vi "Settings Dialog.vi"(8 "error in (no error)":errorcluster caption="错误输入（无错误）", 11 "Configuration in":T1={"Hardware Configuration"={"Physical Channel"="", "Maximum Input"=0.0, "Minimum Input"=0.0, "Sample Rate"=0.0, "Number of Samples"=0}, "Analysis Configuration"={"Statistics"=TRUE}, "New Data Behavior"=enum."Replace", "HWInfo"=""} caption="配置输入") -> (0 "error out":errorcluster caption="错误输出", 2 "UI Refresh Needed?":bool caption="需要刷新UI？", 3 "Configuration out":T1={"Hardware Configuration"={"Physical Channel"="", "Maximum Input"=0.0, "Minimum Input"=0.0, "Sample Rate"=0.0, "Number of Samples"=0}, "Analysis Configuration"={"Statistics"=TRUE}, "New Data Behavior"=enum."Replace", "HWInfo"=""} caption="配置输出")   [LabVIEW 2014, in "Acquisitions.lvlib"]
doc: "用于选择用户设置的对话框。"
uses:
  Acquisitions.lvlib
  User Specified Data.ctl
  HW Configuration.ctl
  AcqControls/Analysis Configuration.ctl
  AcqControls/New Data Behavior.ctl
panel:
  in  "采集模块编号":string
  in  "Number of Samples":i32=1000 caption="采样数"
  in  "Sample Rate":dbl=1000.0 caption="采样率"
  in  "Minimum Input":dbl=-10.0 caption="最小输入"
  in  "Maximum Input":dbl=10.0 caption="最大输入"
  in  "Physical Channel":tag="Dev1/ai0:31" caption="物理通道"
  in  "New Data Behavior":u16(ring) caption="新采集到数据时如何操作" items=["替换", "叠加", "添加"]
  in  "Cancel Button":bool caption="取消按钮"
  in  "OK Button":bool caption="确定按钮"
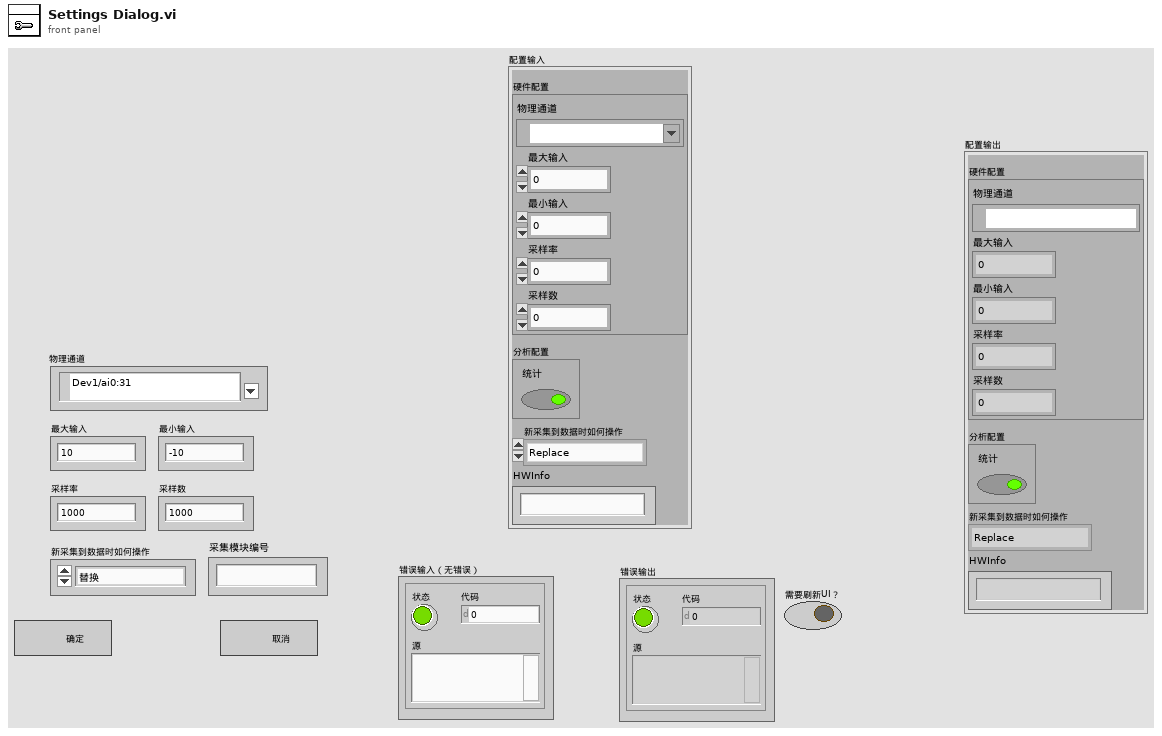
[diagram p1: front panel]
types:
  T1 = typedef "Acquisitions.lvlib/User Specified Data.ctl" = cluster{"Hardware Configuration":T2, "Analysis Configuration":T3, "New Data Behavior":T4, "HWInfo":string}
  T2 = typedef "Acquisitions.lvlib/HW Configuration.ctl" = cluster{"Physical Channel":tag, "Maximum Input":dbl, "Minimum Input":dbl, "Sample Rate":dbl, "Number of Samples":i32}
  T3 = typedef "Acquisitions.lvlib/Analysis Configuration.ctl" = cluster{"Statistics":bool}
  T4 = typedef "Acquisitions.lvlib/New Data Behavior.ctl" = enum16{"Replace", "Overlay", "Append"}
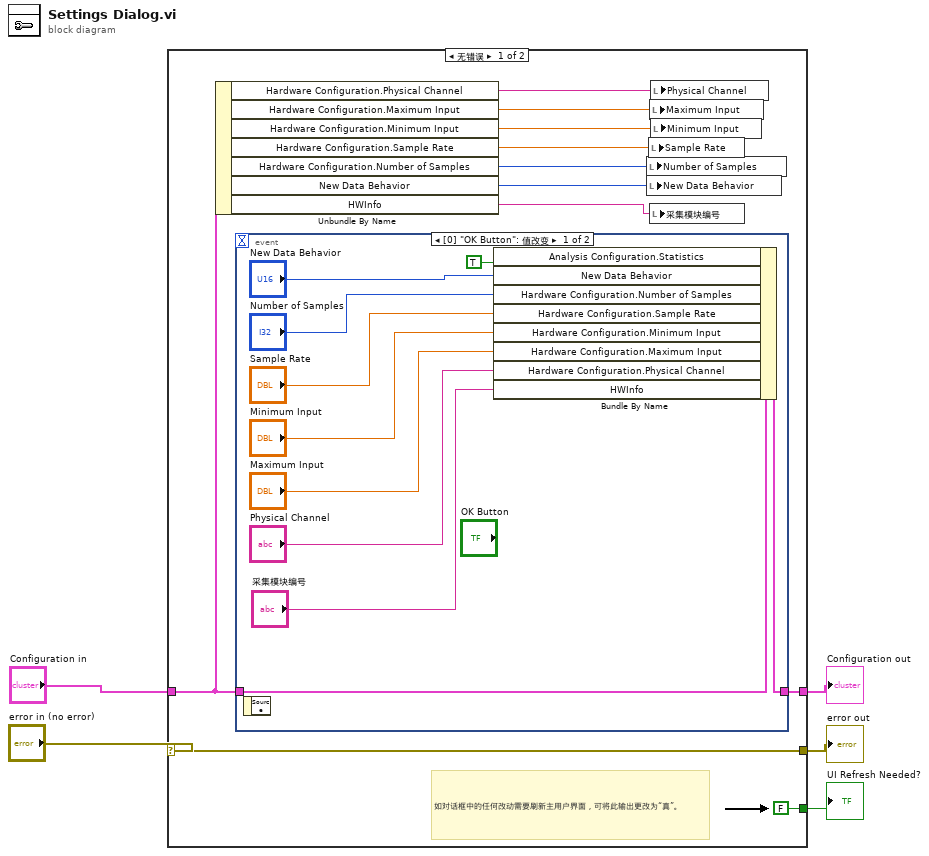
[diagram p0: block diagram]
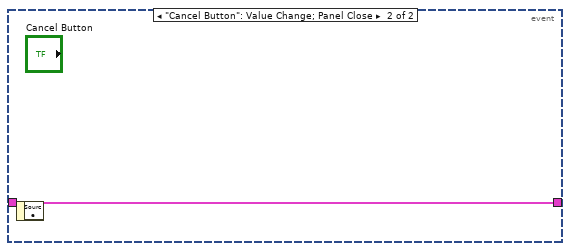
[diagram p2: hidden frame]
diagram:
  n1 = case shown="无错误" "error in (no error)" {
    selector: "error in (no error)" -> [w14 w29]
    tunnel: [w14 w29] -> w4
    tunnel: "Configuration in" -> [w13 w28]
    tunnel: [w16 w28] -> w2
    tunnel: [FALSE ("UI Refresh Needed?") _] -> w1
    frame No Error {
      # "如对话框中的任何改动需要刷新主用户界面，可将此输出更改为“真”。"
      n2 = Unbundle By Name(w13) -> ("Hardware Configuration.Physical Channel"=w12:tag, "Hardware Configuration.Maximum Input"=w11:dbl, "Hardware Configuration.Minimum Input"=w10:dbl, "Hardware Configuration.Sample Rate"=w9:dbl, "Hardware Configuration.Number of Samples"=w8:i32, "New Data Behavior"=w7:T4, "HWInfo"=w6:string)
      n3 = event shown="[0] \"OK Button\": 值改变" {
        selector: _ -> [_ _]
        dyn-events: _ -> [_ _]
        timeout: _ -> [_ _]
        tunnel: [w26 w27] -> w16
        tunnel: w13 -> [w24 w27]
        event "OK Button": Value Change {
          n4 = event-data() -> ()  [unwired: 1 in, 1 out]
          n5 = Bundle By Name(cluster=w24, "Analysis Configuration.Statistics"=TRUE, "New Data Behavior"="New Data Behavior", "Hardware Configuration.Number of Samples"="Number of Samples", "Hardware Configuration.Sample Rate"="Sample Rate", "Hardware Configuration.Minimum Input"="Minimum Input", "Hardware Configuration.Maximum Input"="Maximum Input", "Hardware Configuration.Physical Channel"="Physical Channel", "HWInfo"="采集模块编号") -> (w26:T1)
        }
        event "Cancel Button": Value Change; Panel Close {
          n6 = event-data() -> ()  [unwired: 1 in, 1 out]
        }
      }
      n7 = local write "Number of Samples"(w8) -> ()
      n8 = local write "New Data Behavior"(w7) -> ()
      n9 = local write "Sample Rate"(w9) -> ()
      n10 = local write "Maximum Input"(w11) -> ()
      n11 = local write "采集模块编号"(w6) -> ()
      n12 = local write "Physical Channel"(w12) -> ()
      n13 = local write "Minimum Input"(w10) -> ()
    }
    frame Error {
    }
  }
  "UI Refresh Needed?" <- w1
  "error out" <- w4
  "Configuration out" <- w2
